vi "set_temperature.vi"(8 "error in (no error)":errorcluster, 9 "temperature":dbl, 10 "channel":u8, 11 "LakeShore336 in":refnum<class "Lakeshore_336.lvclass">) -> (0 "error out":errorcluster, 3 "LakeShore336 out":refnum<class "Lakeshore_336.lvclass">)   [LabVIEW 2018, in "Lakeshore_336.lvclass"]
doc: "writes the set temperature of the \"channel\" to the actual instrument"
uses:
  Lakeshore_336.lvclass
  instrument.lvclass
  Drivers/Lake Shore 336/Lake Shore 336.lvlib
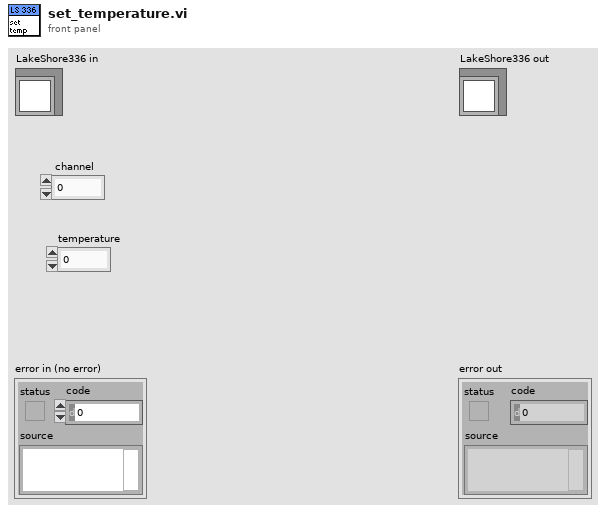
[diagram p1: front panel]
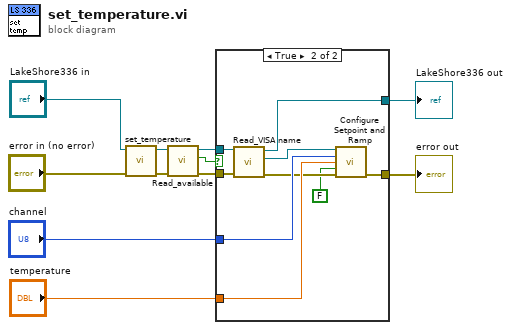
[diagram p0: block diagram]
diagram:
  n1 = call-parent "set_temperature.vi"("error in (no error)"="error in (no error)", "instrument in"="LakeShore336 in") -> ("error out"=w4:errorcluster, "instrument out"=w5:refnum<class "Lakeshore_336.lvclass">)  [unwired: 8 in]
  n2 = call-dynamic "Read_available.vi"("error in (no error)"=w4, "instrument in"=w5) -> ("error out"=w2:errorcluster, "available?"=w1:bool, "instrument out"=w3:refnum<class "Lakeshore_336.lvclass">)  [unwired: 7 in]
  n3 = case shown="True" w1 {
    tunnel: "channel" -> [_ w21]
    tunnel: "temperature" -> [_ w20]
    tunnel: [w13 w19] -> w7
    tunnel: [w12 w18] -> w6
    tunnel: w3 -> [w13 w15]
    tunnel: w2 -> [w12 w14]
    frame False {
    }
    frame True {
      n4 = call-dynamic "Read_VISA name.vi"("error in (no error)"=w14, "instrument in"=w15) -> ("error out"=w17:errorcluster, "VISA resource name"=w22:refnum<visa-resource-name>, "instrument out"=w19:refnum<class "Lakeshore_336.lvclass">)  [unwired: 7 in]
      n5 = call "Configure Setpoint and Ramp.vi"("VISA resource name"=w22, "Output's Control Loop (1:1)"=w21, "Setpoint (0.00000)"=w20, "Setpoint Ramping \nEnable (F: Off)"=FALSE ("Setpoint Ramping \nEnable (F: Off)"), "error in (no error)"=w17) -> ("error out"=w18:errorcluster)  [unwired: 9 in, 1 out]
    }
  }
  "error out" <- w6
  "LakeShore336 out" <- w7
